vi "test_VIRefnumScalar.vi"(8 "error in (no error)":errorcluster) -> (0 "error out":errorcluster)   [LabVIEW 2013]
uses:
  Run Test (VIRefnum Scalar).vi
  Caraya.lvlib
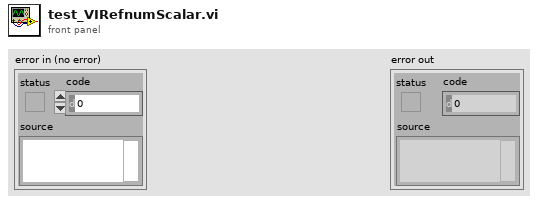
[diagram p1: front panel]
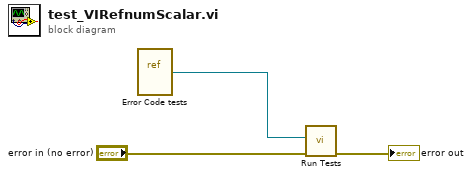
[diagram p0: block diagram]
diagram:
  n1 = vi-ref "Error Code tests.vi"() -> (w1:refnum<vi>)
  n2 = call-poly "Run Tests.vi"("error in"="error in (no error)", "VI Refnum"=w1) -> ("error out"=→"error out":errorcluster)  [unwired: 9 in]
